vi "BGA244_Global.vi"() -> ()   [LabVIEW 2019]
panel:
  out "BGA244_ST":u32(colorbox)
  out "BGA244_Purity":dbl
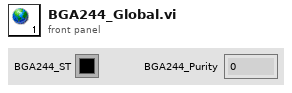
[diagram p1: front panel]
diagram:
